vi "Write Interlock_Enable.vi"(8 "error in":errorcluster, 10 "INTLK_Enable":bool, 11 "IF_XX in":refnum<class "IF_XX.lvclass">) -> (0 "error out":errorcluster, 3 "IF_XX out":refnum<class "IF_XX.lvclass">)   [LabVIEW 2019, in "IF_XX.lvlib" / "IF_XX.lvclass"]
uses:
  Library/IF_XX.lvclass
  C:/Users/Public/Documents/Development/builds/Engine/Monitored Actor.lvlibp/Monitored Actor/Monitored Actor/Monitored Actor.lvclass
  C:/Users/Public/Documents/Development/builds/Instruments/Instruments.lvlibp/Library/Instruments.lvclass
  builds/Engine/Monitored Actor.lvlibp/Monitored Actor/Monitored Actor/Read Actor Label.vi
  builds/Instruments/Instruments.lvlibp/Accessors/Generate Warning.vi
  builds/Instruments/PowerSupply.lvlibp/Library/PowerSupply.lvclass
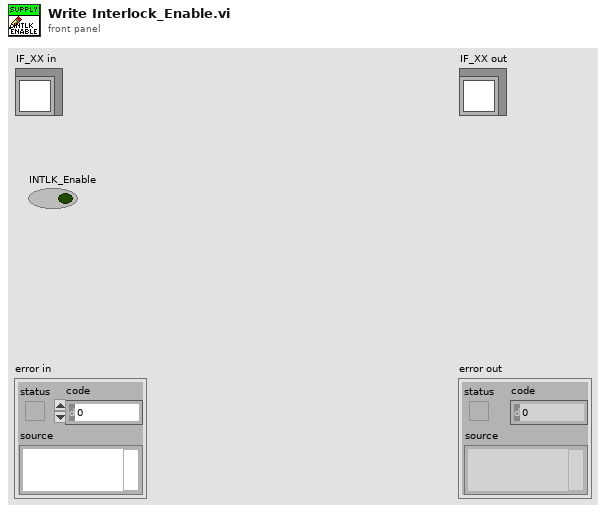
[diagram p1: front panel]
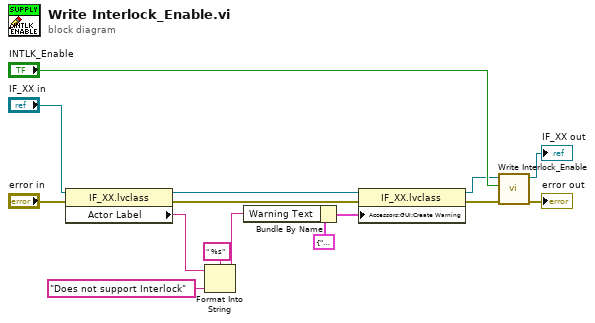
[diagram p0: block diagram]
diagram:
  n1 = property class="IF_XX.lvclass"(reference="IF_XX in", error in="error in") -> (reference out=w6:refnum<class "IF_XX.lvclass">, error out=w5:errorcluster, "Actor Label"=w9:string)
  n2 = Format Into String(format string=" %s", initial string=w9, "Does not support Interlock" ("input 1")) -> (resulting string=w12:string)  [unwired: 1 in, 1 out]
  n3 = Bundle By Name(cluster=cluster{"Warning Text":string, "code":i32} {"Warning Text"="", "code"=5000008} ("Create Warning"), "Warning Text"=w12) -> (w8:cluster{"Warning Text":string, "code":i32})
  n4 = property class="IF_XX.lvclass"(reference=w6, error in=w5, "Accessors:GUI:Create Warning"=w8) -> (reference out=w1:refnum<class "IF_XX.lvclass">, error out=w2:errorcluster)
  n5 = call-parent "Write Interlock_Enable.vi"("error in"=w2, "INTLK_Enable"="INTLK_Enable", "PowerSupply in"=w1) -> ("error out"=→"error out":errorcluster, "PowerSupply out"=→"IF_XX out":refnum<class "IF_XX.lvclass">)  [unwired: 7 in]
